vi "GetSuccessors.vi"(8 "error in (no error)":errorcluster, 10 "AbstractMapNode Ref":refnum<data-value>, 11 "WorldMap in":refnum<class "NI_Robotics_OccupancyGridWorldMap.lvclass">) -> (0 "error out":errorcluster, 1 "EdgeCost":dbl[](array[numeric]), 2 "Successors":refnum<data-value>[](array[refnum]), 3 "WorldMap out":refnum<class "NI_Robotics_OccupancyGridWorldMap.lvclass">)   [LabVIEW 2017, in "NI_Robotics_OccupancyGridWorldMap.lvclass"]
uses:
  <vilib>/robotics/Navigation/shared/WorldMap/OccupancyGridWorldMap/NI_Robotics_OccupancyGridWorldMap.lvclass
  <vilib>/robotics/Navigation/shared/MapNode/AbstractMapNode/NI_Robotics_AbstractMapNode.lvclass
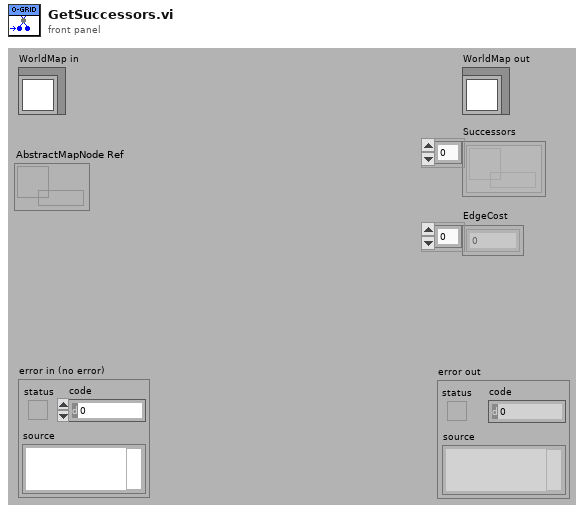
[diagram p1: front panel]
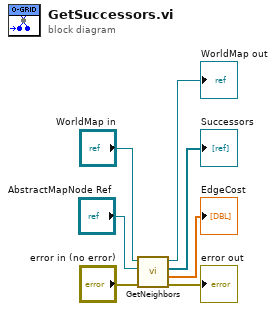
[diagram p0: block diagram]
diagram:
  n1 = call <vilib>:"GetNeighbors.vi"("error in (no error)"="error in (no error)", "AbstractMapNode Ref"="AbstractMapNode Ref", "WorldMap in"="WorldMap in") -> ("error out"=→"error out":errorcluster, "EdgeCost"=→"EdgeCost":dbl[], "Successors"=→"Successors":refnum<data-value>[], "WorldMap out"=→"WorldMap out":refnum<class "NI_Robotics_OccupancyGridWorldMap.lvclass">)  [unwired: 5 in]
